vi "Keithley 6514 Current Example.vi"() -> ()   [LabVIEW 2014, in "KE6514Driver.lvlib"]
uses:
  KE6514Driver.lvlib
panel:
  out "error out":T1
  out "Data Plot":sgl[](graph)
  out "Data":sgl[][](array[numeric]) format="%^.4e"
  in  "Timeout (msecs)":u32=5000
  in  "Trigger Delay":sgl min=0 max=999.9999 step=0.0001 format="%.2f"
  in  "Trigger Count":i16=10 min=1 max=2500 step=1
  in  "Autorange Lower Limit (V)":sgl=2.1 min=0 max=210 step=0.1 format="%^.2e"
  in  "Autorange Upper Limit (V)":sgl=210.0 min=0 max=210 step=0.1 format="%^.2e"
  in  "External Feedback Enabled?":bool
  in  "Driven Guard?":bool
  in  "Check For SCPI Errors?":bool=TRUE
  in  "Range Value (V)":sgl=21.0 min=0 max=210 step=0.1 format="%.2f"
  in  "Ranging Method":u16(ring) items=["autorange", "set min range", "set max range", "set range value"]
  in  "Integration Time (NPLCs)":dbl=1.0 min=0.01 max=10.0 step=0.01 format="%.2f"
  in  "Resource":refnum<visa-resource-name>
  # "Input"
  # "Output"
  # "Measurement\n(V)"
  # "Timestamp\n(secs)"
  # "Status"
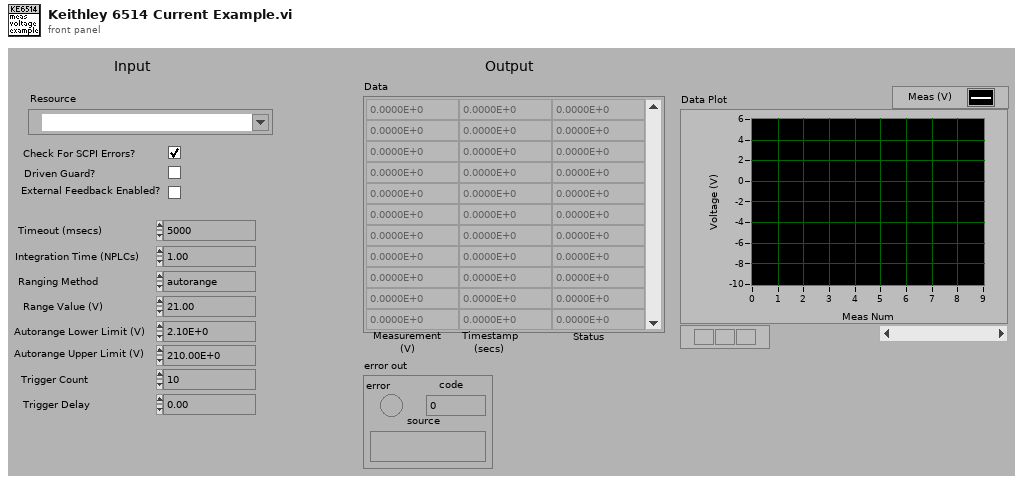
[diagram p1: front panel]
types:
  T1 = cluster{"error":bool, "code":i32, "source":string}
  T2 = cluster{"Read Term Char":enum16{"CR", "LF", "CR + LF", "LF + CR"}, "Baud Rate":enum16{"300", "600", "1200", "2400", "4800", "9600", "19200", "38400", "57600"}, "Flow Control\n(XON / XOFF)":enum16{"Off", "On"}}
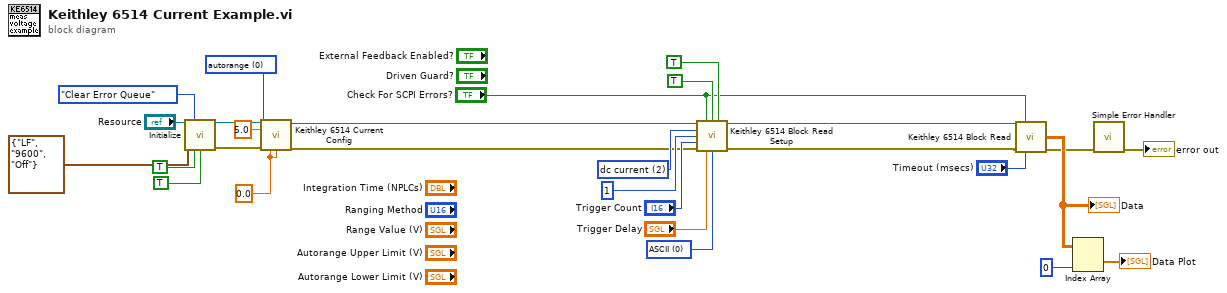
[diagram p0: block diagram]
diagram:
  w2 = 0.0 ("Autorange Upper Limit (A) (21e-3)")
  w3 = u16 0 items=["autorange", "set min range", "set max range", "set range value"] ("range (autorange:0)")
  w16 = u16 0 items=["ASCII", "Single Precision REAL"] ("Data Type (ASCII:0)")
  w22 = u16 2 items=["dc voltage", "resistance", "dc current", "charge"] ("function (Vdc:1)")
  n1 = call "Initialize.vi"("VISA resource name"="Resource", "Error Queue Option"=enum16{"Clear Error Queue", "Error Query"}."Clear Error Queue", "RS-232 Settings"=T2 {"Read Term Char"=enum."LF", "Baud Rate"=enum."9600", "Flow Control\n(XON / XOFF)"=enum."Off"}, "ID Query? (T)"=TRUE, "Reset? (T)"=TRUE) -> ("VISA resource name out"=w6:refnum<visa-resource-name>, "error out"=w7:errorcluster)  [unwired: 1 in, 8 out]
  n2 = call "Keithley 6514 Current Config.vi"("Resource In"=w6, "NPLC value (1.0)"=5.0, "range (autorange:0)"=w3, "error in (no error)"=w7, "Autorange Upper Limit (A) (21e-3)"=w2, "Autorange Lower Limit (A) (21e-12)"=w2) -> ("Resource Out (dupl)"=w5:refnum<visa-resource-name>, "error out"=w4:T1)  [unwired: 3 in, 5 out]
  n3 = call "Keithley 6514 Block Read Setup.vi"("Resource In"=w5, "Check For SCPI Errors? (T)"="Check For SCPI Errors?", "Time (F)"=TRUE, "Status (F)"=TRUE, "function (Vdc:1)"=w22, "Arm Layer Count (1)"=i16 1, "Trigger Layer Count (1)"="Trigger Count", "error in (no error)"=w4, "Trigger Layer Delay (0 secs)"="Trigger Delay", "Data Type (ASCII:0)"=w16) -> ("Resource Out (dupl)"=w15:refnum<visa-resource-name>, "error out"=w14:T1)  [unwired: 4 out]
  n4 = call "Keithley 6514 Block Read.vi"("Resource In"=w15, "Check For SCPI Errors? (T)"="Check For SCPI Errors?", "error in (no error)"=w14, "Timeout (5000 msecs)"="Timeout (msecs)") -> ("Test Data"=w13:sgl[][], "error out"=w10:T1)  [unwired: 10 out]
  "Data" <- w13
  n5 = Index Array(array=w13, index (col)=0 ("disabled index (col)")) -> (element=→"Data Plot":sgl[])  [unwired: 1 in]
  n6 = call <vilib>:"Simple Error Handler.vi"("error in (no error)"=w10) -> ("error out"=→"error out":errorcluster)  [unwired: 1 in, 7 out]
